vi "ArmDevices.vi"(4 "error in":errorcluster, 6 "Digitizer Info":T1, 7 "Generator Info":T3) -> (0 "error out":errorcluster, 2 "Digitizer Info Out":T1, 3 "Generator Info Out":T3)   [LabVIEW 2018]
uses:
  Controls/GeneratorInfo.ctl
  <vilib>/userdefined/High Color/nirio_resource_hc.ctl
  Controls/DigitizerInfo.ctl
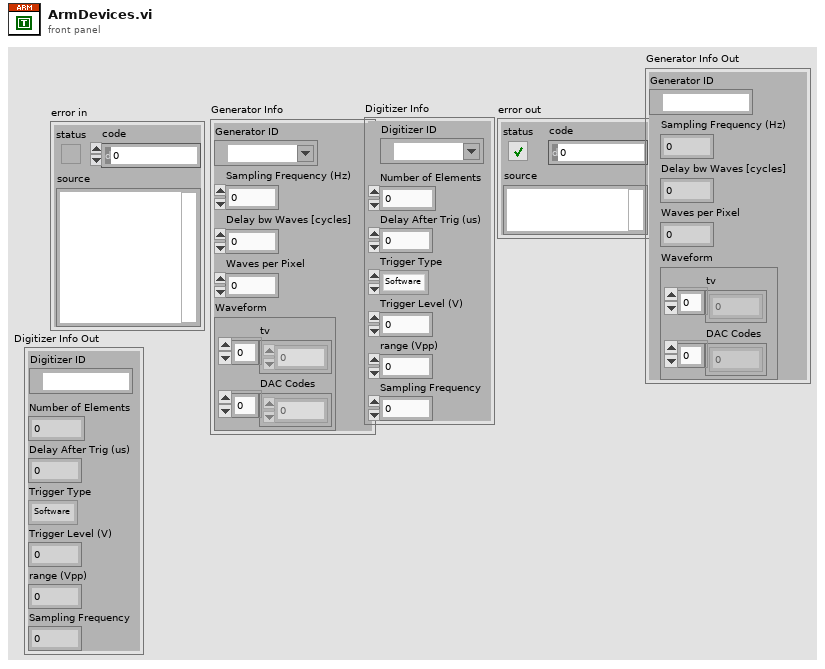
[diagram p1: front panel]
types:
  T1 = typedef "DigitizerInfo.ctl" = cluster{"Digitizer ID":T2, "Number of Elements":u16, "Delay After Trig (us)":dbl, "Trigger Type":enum8{"Software", "Data Edge"}, "Trigger Level (V)":dbl, "range (Vpp)":dbl, "Sampling Frequency":dbl}
  T2 = typedef "nirio_resource_hc.ctl" = tag
  T3 = typedef "GeneratorInfo.ctl" = cluster{"Generator ID":T2, "Sampling Frequency (Hz)":u64, "Delay bw Waves [cycles]":u16, "Waves per Pixel":u32, "Waveform":cluster{"tv":dbl[], "DAC Codes":u16[]}}
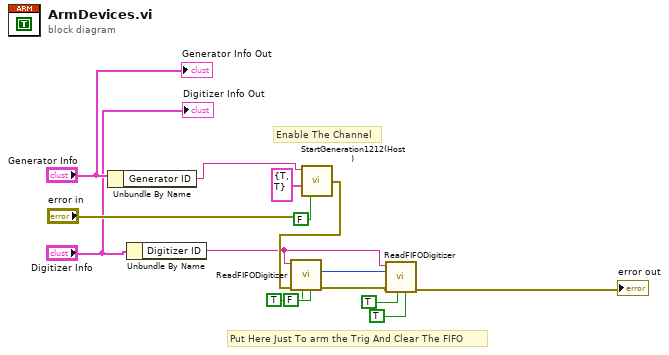
[diagram p0: block diagram]
diagram:
  # "Enable The Channel"
  # "Put Here Just To arm the Trig And Clear The FIFO"
  n1 = Unbundle By Name("Generator Info") -> ("Generator ID"=w13:T2)
  n2 = Unbundle By Name("Digitizer Info") -> ("Digitizer ID"=w5:T2)
  n3 = call "StartGeneration1212(Host).vi"("SYNC"=FALSE, "Channel Cluster"=cluster{"CH1 ON ":bool, "CH2 ON":bool} {"CH1 ON "=TRUE, "CH2 ON"=TRUE}, "error in"="error in", "resource name"=w13) -> ("error out"=w10:errorcluster)
  n4 = call "ReadFIFODigitizer.vi"("Read/nElement Count"=FALSE, "Arm Trigger"=TRUE, "error in"=w10, "resource name"=w5) -> ("error out"=w8:errorcluster, "Elements Remaining"=w6:u32)  [unwired: 4 in, 2 out]
  n5 = call "ReadFIFODigitizer.vi"("Read/nElement Count"=TRUE, "Arm Trigger"=TRUE, "error in"=w8, "Number of Elements"=w6, "resource name"=w5) -> ("error out"=→"error out":errorcluster)  [unwired: 3 in, 3 out]
  "Generator Info Out" <- "Generator Info"
  "Digitizer Info Out" <- "Digitizer Info"
